vi "New Value Reference Transport.vi"(7 "Return Error If Unwritten? (T)":bool=TRUE, 10 "Initial Value":variant) -> (0 "error out":errorcluster, 3 "ValueReferenceTransport":refnum<class "ValueReferenceTransport.lvclass">)   [LabVIEW 2017, in "Transport.lvlib" / "ValueReferenceTransport.lvclass"]
doc: "<License>\nCopyright © 2017 Composed Systems, LLC | All rights reserved\nwww.composed.io\n\nAuthor: Ethan Stern <ethan.stern@composed.io>\n\nThis software is provided \"AS IS\" WITHOUT WARRANTIES, either express or implied, AND IS FOR EDUCATIONAL PURPOSES ONLY.\n</License>"
uses:
  ValueReferenceTransport.lvclass
  ValueReferenceTransport.lvclass/ValueReferenceTransport.ctl
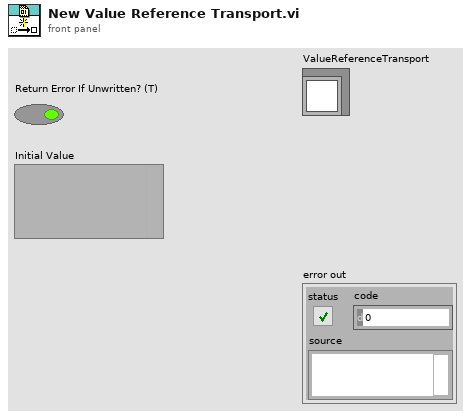
[diagram p1: front panel]
types:
  T1 = cluster{"Data":variant, "Publication Time":timestamp}
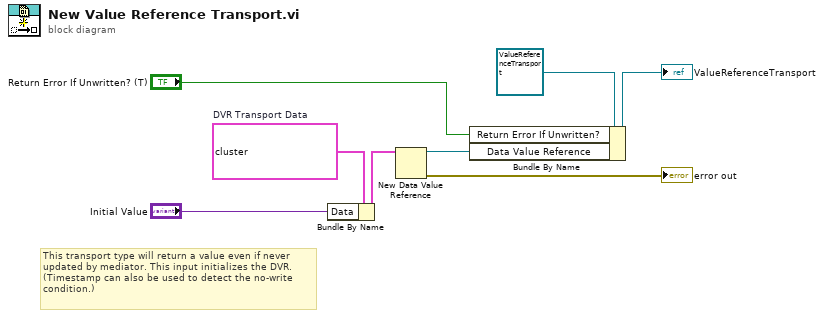
[diagram p0: block diagram]
diagram:
  w5 = T1 {"Data"=variant, "Publication Time"=timestamp(0 s since 1904-01-01)}  # DVR Transport Data
  # "This transport type will return a value even if never\nupdated by mediator. This input initializes the DVR.\n(Timestamp can also be used to detect the no-write\ncondition.)"
  n1 = Bundle By Name(cluster=w5, "Data"="Initial Value") -> (w3:T1)
  n2 = New Data Value Reference(data value=w3) -> (data value reference=w4:refnum<data-value>, error out=→"error out":errorcluster)  [unwired: 1 in]
  n3 = Bundle By Name(cluster=refnum<class "ValueReferenceTransport.lvclass"> refnum ("TerminalBinding in"), "Return Error If Unwritten?"="Return Error If Unwritten? (T)", "Data Value Reference"=w4) -> (→"ValueReferenceTransport":refnum<class "ValueReferenceTransport.lvclass">)
